vi "programmically take screen shot.vi"() -> ()   [LabVIEW 2020]
uses:
  <vilib>/numeric/Random Number (Range) U64.vi
  <vilib>/numeric/sub_Random U32.vi
panel:
  out "Waveform Chart":u64(graph)
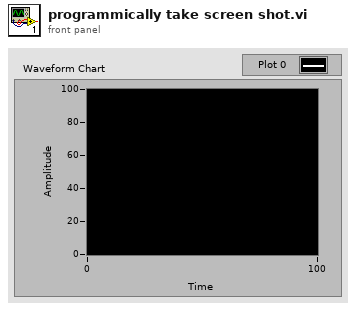
[diagram p1: front panel]
types:
  T1 = typedef "imagedata.ctl" = cluster{"image type":i32, "image depth":i32, "image":u8[], "mask":u8[], "colors":u32[], "Rectangle":cluster{"left":i16, "top":i16, "right":i16, "bottom":i16}}
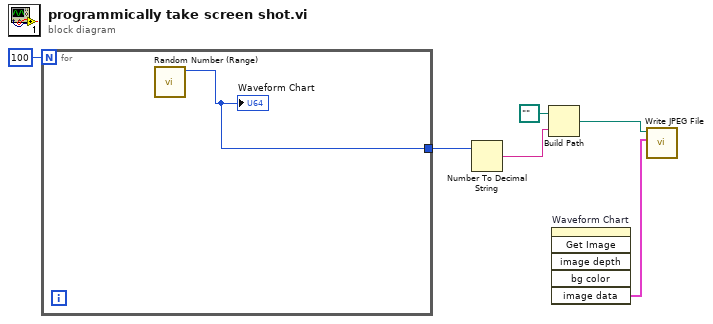
[diagram p0: block diagram]
diagram:
  n1 = for {
    N: 100 -> [_]
    tunnel: [w7] -> w5
    n2 = call-poly <vilib>:"Random Number (Range).vi"() -> ("number"=w7:u64)  [unwired: 11 in]
    "Waveform Chart" <- w7
  }
  n3 = Number To Decimal String(number=w5) -> (decimal integer string=w4:string)  [unwired: 1 in]
  n4 = Build Path(base path=path "", name or relative path=w4) -> (appended path=w2:path)
  n5 = invoke on="Waveform Chart" class="WFChart (strict)" method="Get Image"() -> ("image data"=w3:T1)  [unwired: 6 in, 5 out]
  n6 = call <vilib>:"Write JPEG File.vi"("image data"=w3, "path to JPEG file"=w2) -> ()  [unwired: 8 in, 2 out]
